vi "EMD8216 initial.vi"(7 "TimeOut_ms":u16, 8 "Remote_port":u16, 9 "Host_Port":u16, 10 "IP_Address":u8[](array[numeric]), 11 "CardID":u32) -> (2 "CardType out":u8, 3 "error_code":u32)   [LabVIEW 2015, in "EMD8216_64.lvlib"]
doc: "EMD8216Status EMD8216_initial(u32 CardID,u8 IP_Address[4],u16 Host_Port,u16 Remote_port,u16 TimeOut_ms,u8 *CardType);"
uses:
  EMD8216_64.lvlib
  EMD8216_64.dll
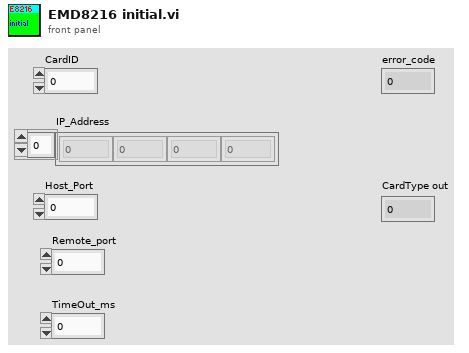
[diagram p1: front panel]
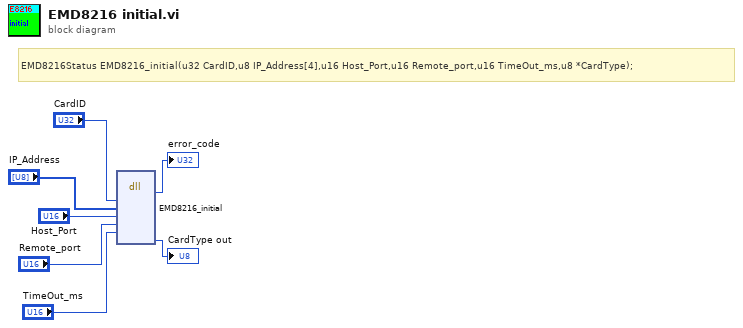
[diagram p0: block diagram]
diagram:
  # "EMD8216Status EMD8216_initial(u32 CardID,u8 IP_Address[4],u16 Host_Port,u16 Remote_port,u16 TimeOut_ms,u8 *CardType);"
  n1 = dll-call lib="C:/Users/jeff.lin.MINAIK/Documents/Soulkai/Labview/io/EMD8216_64/EMD8216_64/EMD8216_64.*" fn="EMD8216_initial"("CardID"="CardID", "IP_Address"="IP_Address", "Host_Port"="Host_Port", "Remote_port"="Remote_port", "TimeOut_ms"="TimeOut_ms") -> ("error_code"=→"error_code":u32, "CardType"=→"CardType out":u8)  [unwired: 9 in, 2 out]
